vi "Create Trigger Model ConfigList Recall Block.vi"(6 "Index Point":i32=1 min=1 max=999999 format="%#.6g", 7 "Enable Index (False)":bool, 8 "error in (no error)":errorcluster, 9 "Configuration List Name":string="SOURCE_LIST", 10 "Block Number (1)":i32=1 min=1 format="%#.6g", 11 "VISA resource name":refnum<visa-resource-name>) -> (0 "error out":errorcluster, 3 "VISA resource name out":refnum<visa-resource-name>)   [LabVIEW 2018, in "Keithley DMM7512.lvlib"]
doc: "This VI recalls the system settings that are stored in a configuration list."
uses:
  <instrlib>/Keithley DMM7512/Keithley DMM7512.lvlib
panel:
  # "True"
  # "False"
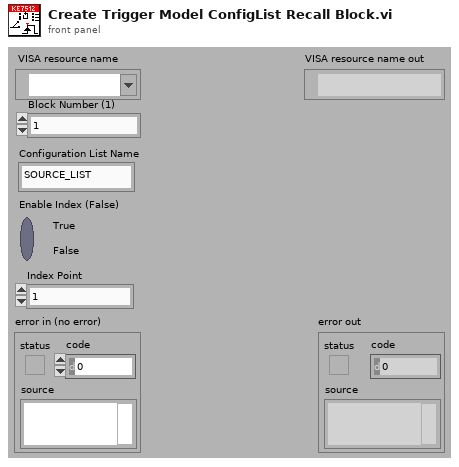
[diagram p1: front panel]
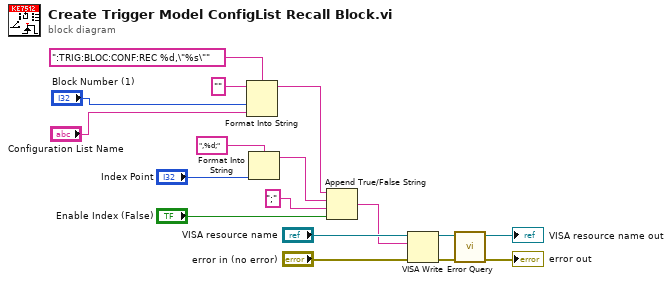
[diagram p0: block diagram]
diagram:
  n1 = Format Into String(format string=":TRIG:BLOC:CONF:REC %d,\"%s\"", initial string="", "Block Number (1)", "Configuration List Name") -> (resulting string=w6:string)  [unwired: 1 in, 1 out]
  n2 = Format Into String(format string=",%d;", "Index Point") -> (resulting string=w4:string)  [unwired: 2 in, 1 out]
  n3 = Append True/False String(1:"Enable Index (False)", 2:";" ("true string"), 3:w4, 4:w6) -> (0:w5:string)
  n4 = VISA Write(VISA resource name="VISA resource name", write buffer=w5, error in (no error)="error in (no error)") -> (VISA resource name out=w13:refnum<visa-resource-name>, error out=w12:errorcluster)  [unwired: 1 out]
  n5 = call <instrlib>:"Error Query.vi"("error in (no error)"=w12, "VISA resource name"=w13) -> ("error out"=→"error out":errorcluster, "VISA resource name out"=→"VISA resource name out":refnum<visa-resource-name>)  [unwired: 8 out]
